vi "Open Excel File.vi"(8 "error in":errorcluster, 10 "file path":path, 11 "excelRefs in":T1) -> (0 "error out":errorcluster, 3 "excelRefs out":T1)   [LabVIEW 2020]
uses:
  Controls/excelRefContainer.ctl
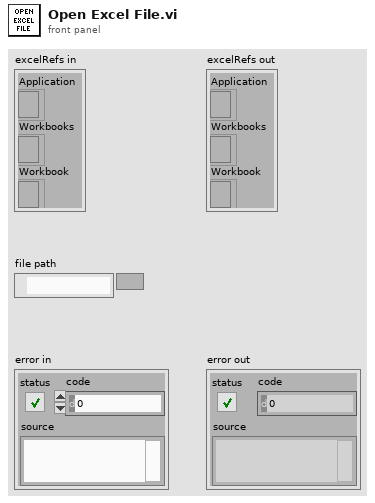
[diagram p1: front panel]
types:
  T1 = typedef "excelRefContainer.ctl" = cluster{"Application":refnum<k7>, "Workbooks":refnum<k7>, "Workbook":refnum<k7>}
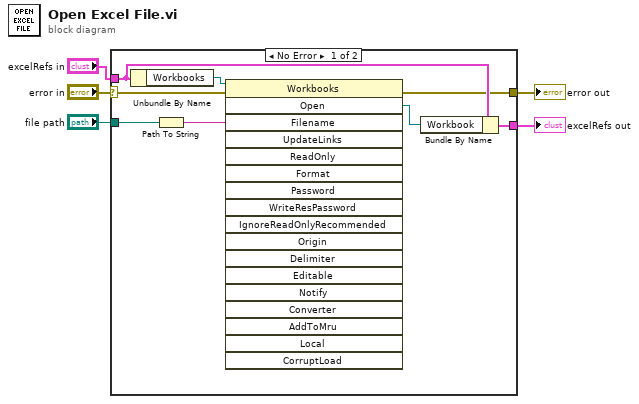
[diagram p0: block diagram]
diagram:
  n1 = case shown="No Error" "error in" {
    selector: "error in" -> [w11 w15]
    tunnel: [w7 w15] -> w4
    tunnel: [w6 w14] -> w3
    tunnel: "excelRefs in" -> [w9 w14]
    tunnel: "file path" -> [w12 _]
    frame No Error {
      n2 = Unbundle By Name(w9) -> ("Workbooks"=w10:refnum<k7>)
      n3 = Path To String(path=w12) -> (string=w13:string)
      n4 = invoke class="Workbooks" method="Open"(reference=w10, error in=w11, "Filename"=w13) -> (error out=w7:errorcluster, "Open"=w8:refnum<k7>)  [unwired: 15 in, 16 out]
      n5 = Bundle By Name(cluster=w9, "Workbook"=w8) -> (w6:T1)
    }
    frame Error {
    }
  }
  "error out" <- w4
  "excelRefs out" <- w3
